vi "round val.vi"(1 "num in":dbl) -> (0 "num out":dbl)   [LabVIEW 2012]
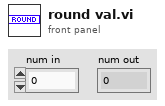
[diagram p1: front panel]
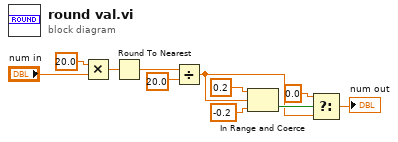
[diagram p0: block diagram]
diagram:
  n1 = Multiply(x=20.0, y="num in") -> (x*y=w8:dbl)
  n2 = Round To Nearest(number=w8) -> (nearest integer value=w7:dbl)
  n3 = Divide(x=w7, y=20.0) -> (x/y=w1:dbl)
  n4 = In Range and Coerce(upper limit=0.2, x=w1, lower limit=-0.2) -> (In Range?=w3:bool)  [unwired: 1 out]
  n5 = Select(t=0.0, s=w3, f=w1) -> (s? t:f=→"num out":dbl)
